vi "Set Callback Events.vi"(8 "error in (no error)":errorcluster, 10 "Callback Events":cluster{}, 11 "SourceGrid in":refnum<class "SourceGrid.lvclass">) -> (0 "error out":errorcluster, 3 "SourceGrid out":refnum<class "SourceGrid.lvclass">)   [LabVIEW 2024]
uses:
  SourceGrid.lvclass/SourceGrid.ctl
  SourceGrid.lvclass
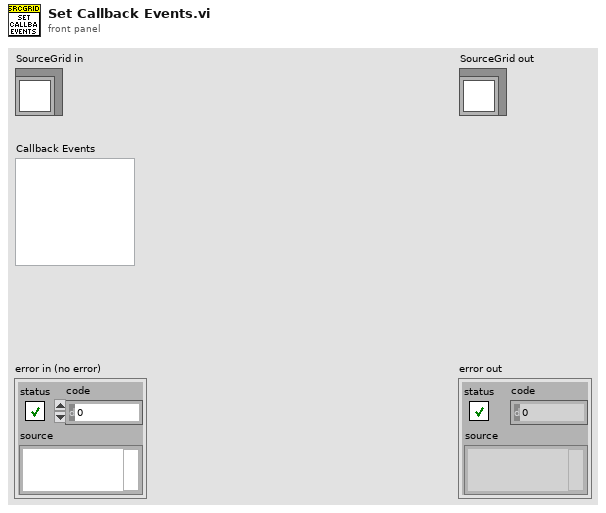
[diagram p1: front panel]
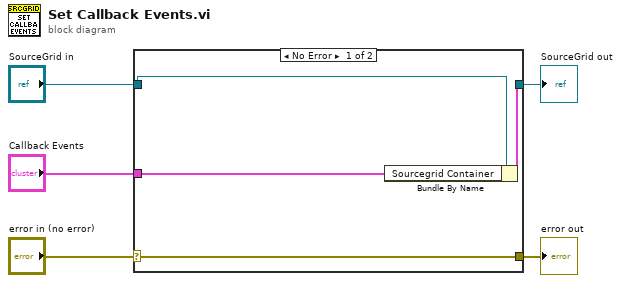
[diagram p0: block diagram]
diagram:
  n1 = case shown="No Error" "error in (no error)" {
    selector: "error in (no error)" -> [w9 w10]
    tunnel: [w9 w10] -> w4
    tunnel: [w7 w11] -> w2
    tunnel: "SourceGrid in" -> [w8 w11]
    tunnel: "Callback Events" -> [w6 _]
    frame No Error {
      n2 = Bundle By Name(cluster=w8, "Sourcegrid Container"=w6) -> (w7:cluster{})
    }
    frame Error {
    }
  }
  "error out" <- w4
  "SourceGrid out" <- w2
